vi "动态调用子vi.vi"(1 "Front Panel Window:State":T1(ring), 2 "error in (no error)":errorcluster, 3 "被调用的子vi":string, 4 "VI Refnum":refnum<vi>) -> (0 "error out":errorcluster)   [LabVIEW 2014]
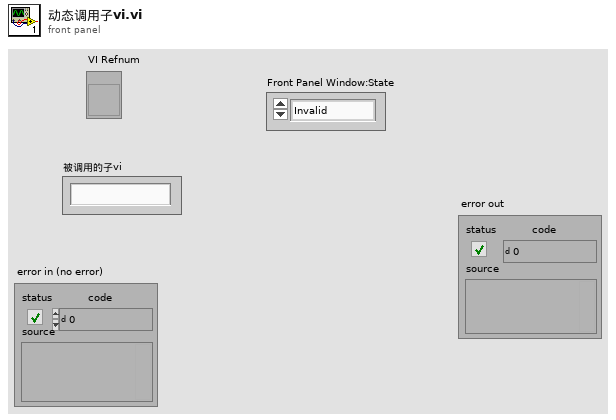
[diagram p1: front panel]
types:
  T1 = enum32{"Invalid", "Standard", "Closed", "Hidden", "Minimized", "Maximized"}
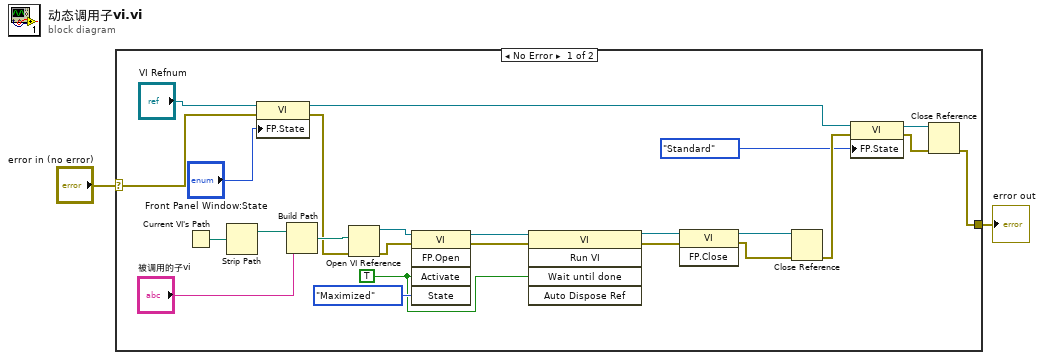
[diagram p0: block diagram]
diagram:
  n1 = case shown="No Error" "error in (no error)" {
    selector: "error in (no error)" -> [w25 w27]
    tunnel: [w7 w27] -> w1
    frame No Error {
      w4 = TRUE ("Activate?")
      n2 = Current VI's Path() -> (path=w24:path)
      n3 = Strip Path(path=w24) -> (stripped path=w23:path)  [unwired: 1 out]
      n4 = property class="VI"(reference="VI Refnum", error in=w25, "FP.State"="Front Panel Window:State") -> (reference out=w11:refnum<vi>, error out=w20:errorcluster)
      n5 = Build Path(base path=w23, name or relative path="被调用的子vi") -> (appended path=w21:path)
      n6 = Open VI Reference(vi path=w21, error in (no error)=w20) -> (vi reference=w19:refnum<vi>, error out=w18:errorcluster)  [unwired: 4 in]
      n7 = invoke class="VI" method="FP.Open"(reference=w19, error in=w18, "Activate"=w4, "State"=T1."Maximized") -> (reference out=w17:refnum<vi>, error out=w16:errorcluster)  [unwired: 1 in, 3 out]
      n8 = invoke class="VI" method="Run VI"(reference=w17, error in=w16, "Wait until done"=w4) -> (reference out=w15:refnum<vi>, error out=w14:errorcluster)  [unwired: 2 in, 3 out]
      n9 = invoke class="VI" method="FP.Close"(reference=w15, error in=w14) -> (reference out=w13:refnum<vi>, error out=w12:errorcluster)  [unwired: 1 in, 1 out]
      n10 = Close Reference(reference=w13, error in (no error)=w12) -> (error out=w10:errorcluster)
      n11 = property class="VI"(reference=w11, error in=w10, "FP.State"=T1."Standard" ("Front Panel Window:State")) -> (reference out=w9:refnum<vi>, error out=w8:errorcluster)
      n12 = Close Reference(reference=w9, error in (no error)=w8) -> (error out=w7:errorcluster)
    }
    frame Error {
    }
  }
  "error out" <- w1
